vi "DCMotors3.vi"(6 "Stop":bool, 8 "error in":errorcluster, 9 "Motors Renum":cluster{"Num":i32, "Directly":bool, "KM":dbl}[](array[cluster])=[{"Num"=1, "Directly"=TRUE, "KM"=0.97}, {"Num"=3, "Directly"=FALSE, "KM"=1.0}, {"Num"=0, "Directly"=FALSE, "KM"=0.98}, {"Num"=2, "Directly"=TRUE, "KM"=1.0}], 10 "Input":dbl[](array[slide])=[0.0, 0.0, -0.01, 0.0] step=1.0 scale=-100.0..100.0, 11 "CAN in":refnum<class "CAN.lvclass">) -> (0 "error out":errorcluster, 3 "CAN out":refnum<class "CAN.lvclass">)   [LabVIEW 2020]
uses:
  <vilib>/High Genius/HG_WSI_Tookit/Dependencies/Library/CAN/CAN.lvclass
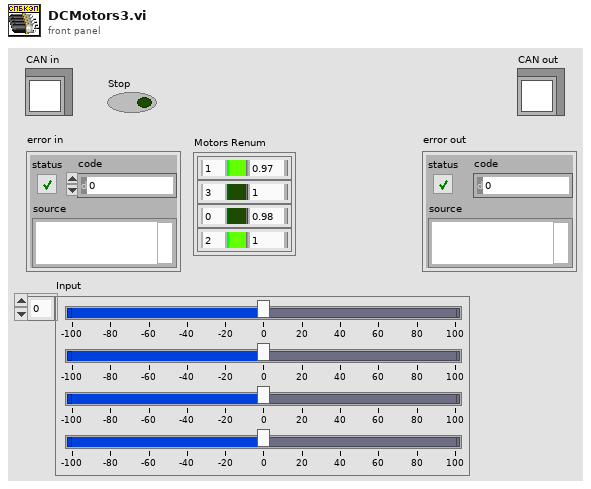
[diagram p1: front panel]
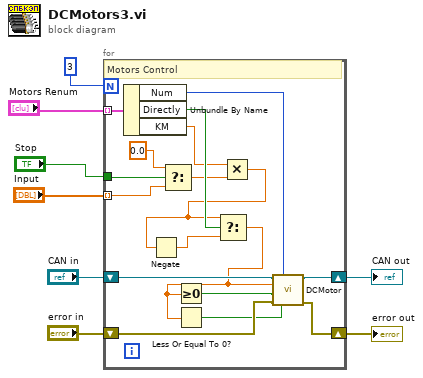
[diagram p0: block diagram]
diagram:
  n1 = for {
    N: 3 -> [_]
    shift-right: [w18] -> w7
    shift-left: "CAN in" -> [w17]
    shift-right: [w14] -> w5
    shift-left: "error in" -> [w15]
    tunnel: "Input" -> [w22] mode=indexing
    tunnel: "Motors Renum" -> [w24] mode=indexing
    tunnel: "Stop" -> [w20]
    # "Motors Control"
    n2 = Unbundle By Name(w24) -> ("Num"=w19:i32, "Directly"=w23:bool, "KM"=w9:dbl)
    n3 = Select(t=0.0, s=w20, f=w22) -> (s? t:f=w10:dbl)
    n4 = Multiply(x=w9, y=w10) -> (x*y=w11:dbl)
    n5 = Negate(x=w11) -> (-x=w25:dbl)
    n6 = Select(t=w11, s=w23, f=w25) -> (s? t:f=w12:dbl)
    n7 = Greater Or Equal To 0?(x=w12) -> (x >= 0?=w16:bool)
    n8 = Less Or Equal To 0?(x=w12) -> (x <= 0?=w13:bool)
    n9 = call "DCMotor.vi"("INB"=w13, "PWM"=w19, "error in (no error)"=w15, "INA"=w16, "Duty Cycle"=w12, "CAN in"=w17) -> ("error out"=w14:errorcluster, "CAN out"=w18:refnum<class "CAN.lvclass">)  [unwired: 4 in]
  }
  "CAN out" <- w7
  "error out" <- w5
